vi "8FM.vi"() -> ()   [LabVIEW 2013]
uses:
  <vilib>/Analysis/NI_AALPro.lvlib
panel:
  out "demodulated signal":dynamicdata(graph)
  out "FM signal":dynamicdata(graph)
  out "carrier signal":dynamicdata(graph)
  in  "FC":dbl=100.0 caption="Frequency"
  in  "AC":dbl=1.0 caption="Amplitude"
  out "beta":dbl
  in  "kf":dbl
  out "message siganl":dynamicdata(graph)
  in  "Am":dbl=1.0 caption="Amplitude"
  in  "Fm":dbl=10.0 caption="Frequency"
  # "FREQUENCY MODULATION"
  # "K MANGARATNAM\n23A91A0429\nECE-A"
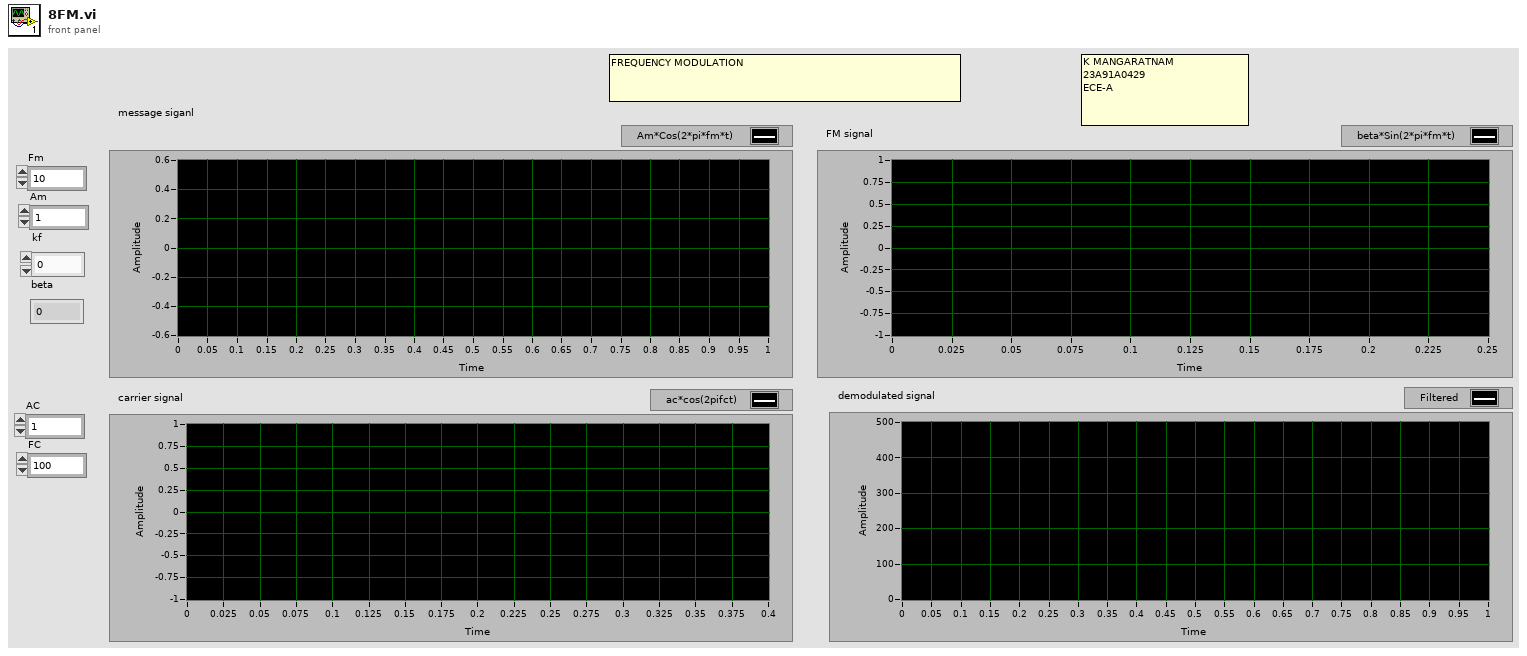
[diagram p1: front panel]
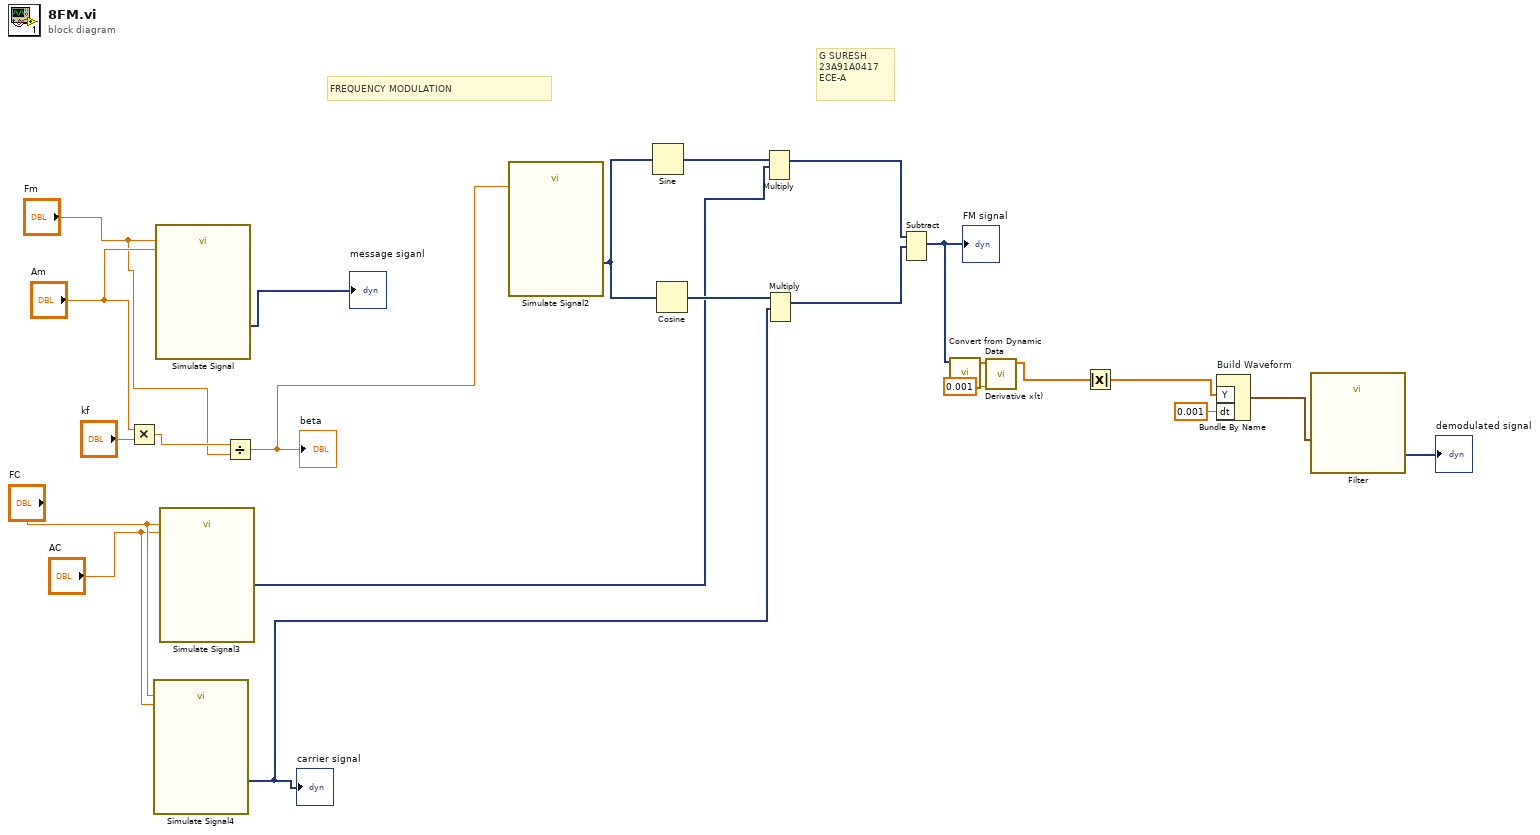
[diagram p0: block diagram]
diagram:
  # "G SURESH\n23A91A0417\nECE-A"
  # "FREQUENCY MODULATION"
  n1 = Multiply(x="Am", y="kf") -> (x*y=w20:dbl)
  n2 = call "Simulate Signal4"("Frequency"="FC", "Amplitude"="AC") -> ("ac*cos(2pifct)"=w9:dynamicdata)  [unwired: 12 in, 1 out]
  "carrier signal" <- w9
  n3 = call "Simulate Signal"("Frequency"="Fm", "Amplitude"="Am") -> ("Am*Cos(2*pi*fm*t)"=→"message siganl":dynamicdata)  [unwired: 12 in, 1 out]
  n4 = call "Simulate Signal3"("Frequency"="FC", "Amplitude"="AC") -> ("ac*sin(2*pi*fc*t)"=w12:dynamicdata)  [unwired: 12 in, 1 out]
  n5 = Divide(x=w20, y="Fm") -> (x/y=w18:dbl)
  "beta" <- w18
  n6 = call "Simulate Signal2"("Amplitude"=w18) -> ("beta*Sin(2*pi*fm*t)"=w17:dynamicdata)  [unwired: 13 in, 1 out]
  n7 = Sine(x=w17) -> (sin(x)=w16:dynamicdata)
  n8 = Cosine(x=w17) -> (cos(x)=w15:dynamicdata)
  n9 = Multiply(1:w12, 2:w16) -> (0:w11:dynamicdata)  [unwired: 1 in, 1 out]
  n10 = Multiply(1:w9, 2:w15) -> (0:w10:dynamicdata)  [unwired: 1 in, 1 out]
  n11 = Subtract(1:w10, 2:w11) -> (0:w8:dynamicdata)  [unwired: 1 in, 1 out]
  "FM signal" <- w8
  n12 = call "Convert from Dynamic Data"("Dynamic Data Type"=w8) -> ("Array"=w7:dbl[])  [unwired: 3 in]
  n13 = call <vilib>:"Derivative x(t).vi"("dt"=0.001, "X"=w7) -> ("dX/dt"=w5:dbl[])  [unwired: 8 in, 1 out]
  n14 = Absolute Value(x=w5) -> (abs(x)=w3:dbl[])
  n15 = Bundle By Name "Build Waveform"("Y"=w3, "dt"=0.001) -> (w2:waveform(dbl))  [unwired: 1 in]
  n16 = call "Filter"("Signal"=w2) -> ("Filtered Signal"=→"demodulated signal":dynamicdata)  [unwired: 9 in, 1 out]
